vi "Switch_PinsToSessions.vi"(8 "error in (no error)":errorcluster, 10 "Pins":string[](array[string]), 11 "Semiconductor Module Context":T1) -> (0 "error out":errorcluster, 1 "Channel Lists":string[](array[string]), 2 "Instrument Sessions":refnum<k15>[](array[refnum]), 3 "Semiconductor Module Context Out":T1, 5 "Pin Query Context":refnum<class "MultiplePinMultipleSessionQueryContext.lvclass">)   [LabVIEW 2014]
uses:
  <vilib>/NI_TestStand_SemiconductorModule/NI_TestStand_Semiconductor_Module.lvlibp/PinMap/General/SemiconductorModuleContext.ctl
  <vilib>/NI_TestStand_SemiconductorModule/NI_TestStand_Semiconductor_Module.lvlibp/PinMap/PinQueryContext/MultiplePinMultipleSessionQueryContext/MultiplePinMultipleSessionQueryContext.lvclass
  <vilib>/NI_TestStand_SemiconductorModule/NI_TestStand_Semiconductor_Module.lvlibp/PinMap/Advanced/Custom Instruments/GetSessionData.vi
  <vilib>/NI_TestStand_SemiconductorModule/NI_TestStand_Semiconductor_Module.lvlibp
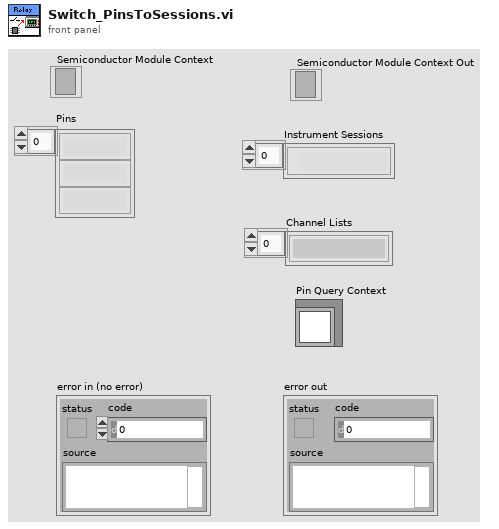
[diagram p1: front panel]
types:
  T1 = typedef "NI_TestStand_Semiconductor_Module.lvlibp/SemiconductorModuleContext.ctl" = refnum<k7>
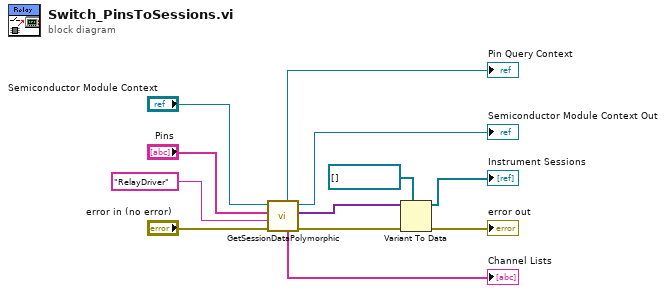
[diagram p0: block diagram]
diagram:
  n1 = call-poly <vilib>:"GetSessionDataPolymorphic.vi"("error in (no error)"="error in (no error)", "Instrument Type Id"="RelayDriver" ("Instrument Type"), "Pins"="Pins", "Semiconductor Module Context"="Semiconductor Module Context") -> ("error out"=w5:errorcluster, "Session Data"=w3:variant[], "Semiconductor Module Context Out"=→"Semiconductor Module Context Out":T1, "Channel Lists"=→"Channel Lists":string[], "Pin Query Context"=→"Pin Query Context":refnum<class "MultiplePinMultipleSessionQueryContext.lvclass">)  [unwired: 2 in, 1 out]
  n2 = Variant To Data(error in=w5, type=refnum<k15>[] [], Variant=w3) -> (data=→"Instrument Sessions":refnum<k15>[], error out=→"error out":errorcluster)
